vi "GetLIDAR.vi"(1 "Roll (deg)":dbl, 2 "Pitch (deg)":dbl, 3 "Raw Horizontal Offset (in)":dbl) -> (0 "LIDAR Distance to Target (in)":dbl)   [LabVIEW 2019]
doc: "This VI converts the raw LIDAR signal into a range in inches and is based on code from FRC 3504. https://www.andymark.com/products/lidar-lite-3"
uses:
  refnums.vi
  GRNF_DIC.vi
  sensors.vi
panel:
  in  "Maximum Pointing Error (deg)":dbl=5.0
  in  "Calibration Offset (in)":dbl=10.0
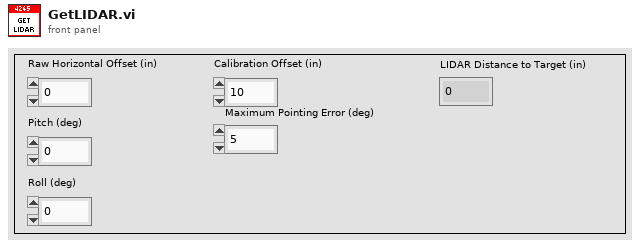
[diagram p1: front panel]
types:
  T1 = typedef "WPI_CounterDevRef.ctl" = cluster{"DevStatus":errorcluster, "CntIndex":T2}
  T2 = typedef "FPGA_CounterCtrSystemIndex.ctl" = enum8{"Ctr 0", "Ctr 1", "Ctr 2", "Ctr 3", "Ctr 4", "Ctr 5", "Ctr 6", "Ctr 7", "Invalid"}
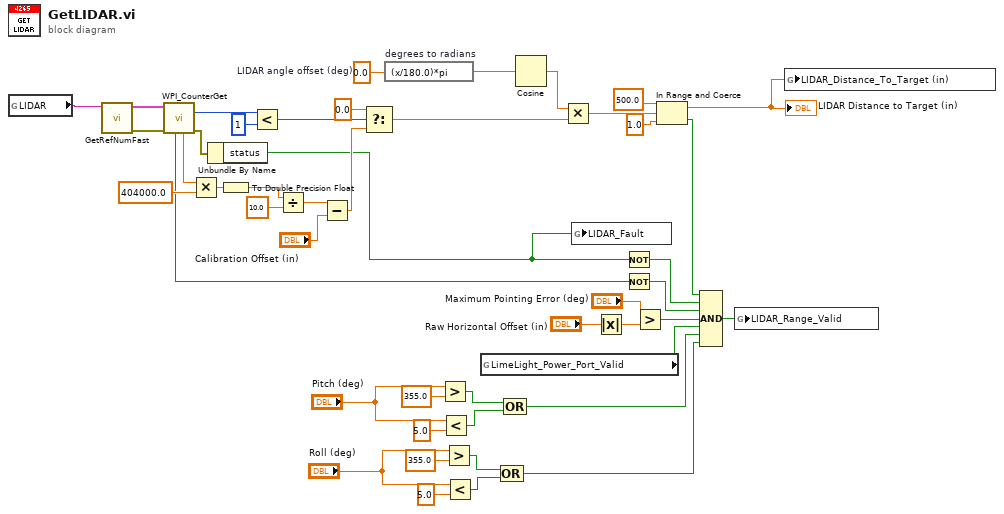
[diagram p0: block diagram]
diagram:
  w3 = 0.0  # LIDAR angle offset (deg)
  n1 = global read "refnums.vi" "LIDAR"() -> (w35:string)
  n2 = call-poly "GetRefNumFast.vi"("RefNum Name"=w35) -> ("Error"=w33:errorcluster, "Device Reference"=w34:T1)  [unwired: 5 in]
  n3 = call <vilib>:"WPI_CounterGet.vi"("error in (no error)"=w33, "CounterDevRef in"=w34) -> ("error out"=w8:errorcluster, "Value"=w44:i32, "Period (sec)"=w37:dbl, "Stopped"=w9:bool)  [unwired: 4 in, 2 out]
  n4 = Multiply(x=w37, y=404000.0) -> (x*y=w43:dbl)
  n5 = Unbundle By Name(w8) -> ("status"=w1:bool)
  n6 = To Double Precision Float(number=w43) -> (double precision float=w42:dbl)
  n7 = Less?(x=w44, y=1) -> (x < y?=w47:bool)
  n8 = Divide(x=w42, y=10.0) -> (x/y=w40:dbl)
  n9 = Subtract(x=w40, y="Calibration Offset (in)") -> (x-y=w38:dbl)
  n10 = Select(t=0.0, s=w47, f=w38) -> (s? t:f=w5:dbl)
  n11 = expression code="(x/180.0)*pi" "degrees to radians"(w3) -> (w2:dbl)
  n12 = Greater?(x="Pitch (deg)", y=355.0) -> (0:w22:bool)
  n13 = Less?(x="Pitch (deg)", y=5.0) -> (x < y?=w21:bool)
  n14 = Greater?(x="Roll (deg)", y=355.0) -> (0:w18:bool)
  n15 = Less?(x="Roll (deg)", y=5.0) -> (x < y?=w17:bool)
  n16 = global read "sensors.vi" "LimeLight_Power_Port_Valid"() -> (w28:bool)
  n17 = Compound Arithmetic op=OR(w18, w17) -> (w13:bool)
  n18 = Compound Arithmetic op=OR(w22, w21) -> (w14:bool)
  n19 = Cosine(x=w2) -> (cos(x)=w6:dbl)
  n20 = Multiply(x=w6, y=w5) -> (x*y=w4:dbl)
  n21 = global write "sensors.vi" "LIDAR_Fault"(w1) -> ()
  n22 = Absolute Value(x="Raw Horizontal Offset (in)") -> (abs(x)=w31:dbl)
  n23 = Not(x=w1) -> (.not. x?=w7:bool)
  n24 = Not(x=w9) -> (.not. x?=w10:bool)
  n25 = Greater?(x="Maximum Pointing Error (deg)", y=w31) -> (0:w29:bool)
  n26 = In Range and Coerce(upper limit=500.0, x=w4, lower limit=1.0 ("x")) -> (coerced(x)=w25:dbl, In Range?=w11:bool)
  "LIDAR Distance to Target (in)" <- w25
  n27 = Compound Arithmetic op=AND(w11, w7, w10, w29, w28, w14, w13) -> (w12:bool)
  n28 = global write "sensors.vi" "LIDAR_Range_Valid"(w12) -> ()
  n29 = global write "sensors.vi" "LIDAR_Distance_To_Target (in)"(w25) -> ()
